vi "SetChannelAutoRange.vi"(2 "On/Off":string, 3 "error out 2":errorcluster, 4 "Channel":string, 5 "reference out 2":refnum<visa-resource-name>) -> (0 "error out":errorcluster, 1 "reference out 3":refnum<visa-resource-name>)   [LabVIEW 2009]
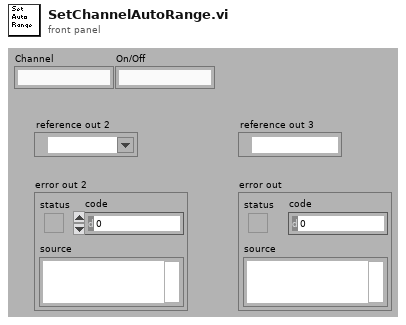
[diagram p1: front panel]
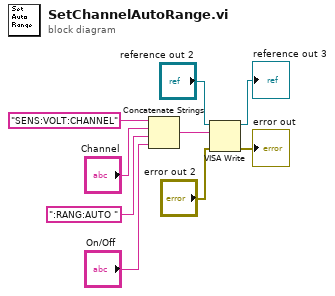
[diagram p0: block diagram]
diagram:
  n1 = Concatenate Strings("SENS:VOLT:CHANNEL" ("write buffer"), "Channel", ":RANG:AUTO " ("string"), "On/Off") -> (w1:string)
  n2 = VISA Write(VISA resource name="reference out 2", write buffer=w1, error in (no error)="error out 2") -> (VISA resource name out=→"reference out 3":refnum<visa-resource-name>, error out=→"error out":errorcluster)  [unwired: 1 out]
